vi "Actor Ref Cache FGV.vi"(6 "Action":T1, 11 "VI Refnum In":refnum<vi>) -> (3 "All Refs Out":refnum<vi>[](array[refnum]))   [LabVIEW 2015]
uses:
  Actor Ref Cache Action.ctl
panel:
  out "size(s)":i32
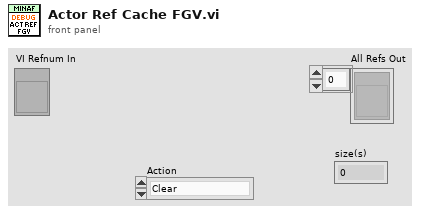
[diagram p1: front panel]
types:
  T1 = typedef "Actor Ref Cache Action.ctl" = enum16{"Clear", "Add Ref", "Remove Ref", "Get All Refs"}
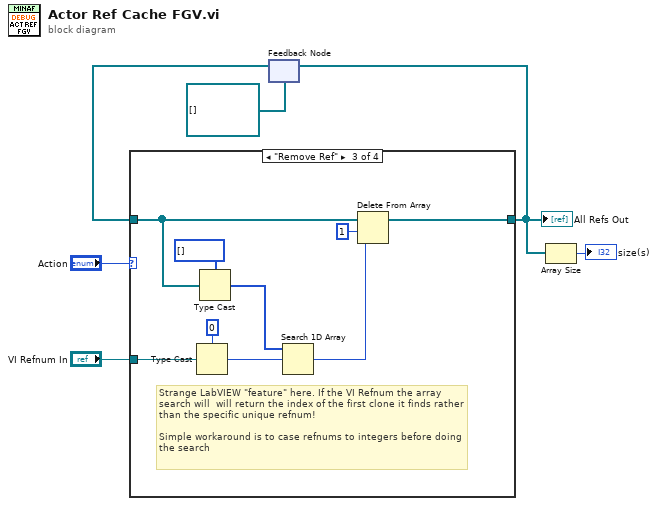
[diagram p0: block diagram]
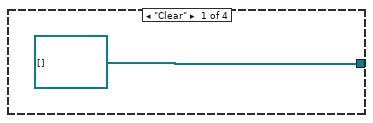
[diagram p2: hidden frame]
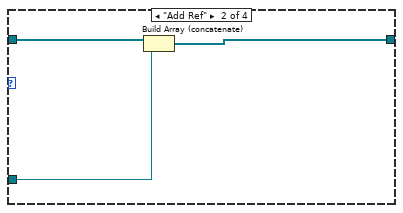
[diagram p3: hidden frame]
diagram:
  n1 = feedback #1(refnum<vi>[] [] ("All Refs Out")) -> (w5:refnum<vi>[])
  n2 = case shown="\"Remove Ref\"" "Action" {
    tunnel: [refnum<vi>[] [] ("All Refs Out") w9 w18 w20] -> w2
    tunnel: w5 -> [_ w10 w16 w20]
    tunnel: "VI Refnum In" -> [_ w8 w13 _]
    frame "Clear" {
    }
    frame "Add Ref" {
      n3 = Build Array (concatenate)(w10, w8) -> (w9:refnum<vi>[])
    }
    frame "Remove Ref" {
      # "Strange LabVIEW \"feature\" here. If the VI Refnum the array search will  will return the index of the first clone it finds rather than the specific unique refnum!\n\nSimple workaround is to case refnums to integers before doing the search"
      n4 = Type Cast(type=0, x=w13) -> (*(type *) &x=w11:i32)
      n5 = Type Cast(type=i32[] [], x=w16) -> (*(type *) &x=w14:i32[])
      n6 = Search 1D Array(1D array=w14, element=w11) -> (index of element=w19:i32)  [unwired: 1 in]
      n7 = Delete From Array(array=w16, length=1, index=w19) -> (array with subset deleted=w18:refnum<vi>[])  [unwired: 1 out]
    }
    frame "Get All Refs" {
    }
  }
  "All Refs Out" <- w2
  n8 = feedback-in #1(w2) -> ()
  n9 = Array Size(array=w2) -> (size(s)=→"size(s)":i32)
